vi "Get Process Variable.vi"(11 "Actuator Cylinder in":refnum<class "Actuator Cylinder.lvclass">) -> (2 "Process Variable":dbl[unit], 3 "Actuator Cylinder out":refnum<class "Actuator Cylinder.lvclass">)   [LabVIEW 2015, in "Actuator Cylinder.lvclass"]
uses:
  Actuator Cylinder.lvclass
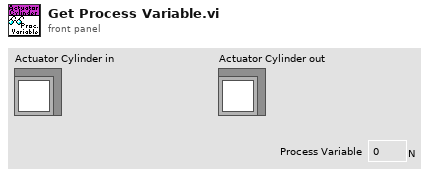
[diagram p1: front panel]
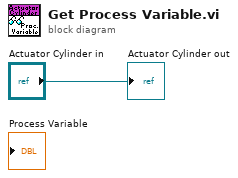
[diagram p0: block diagram]
diagram:
  "Actuator Cylinder out" <- "Actuator Cylinder in"
